vi "ExternalSetParam.vi"(0 "reference":refnum<class "ClassNode.lvclass">, 1 "setParameter":T2, 2 "string":string, 3 "position":T1 {"y" format="%.2f"; "x" format="%.2f"}, 4 "Boolean":bool, 5 "error in (no error)":errorcluster, 7 "ClassPath":path) -> (14 "reference out":refnum<class "ClassNode.lvclass">, 19 "error out":errorcluster)   [LabVIEW 2014, in "ClassNode.lvclass"]
doc: "Sets parameter externaly.\nPossible to set Name,Attrib,Methods and Position"
uses:
  <resource>/Framework/Providers/Open_GDS/UML/ClassNode_class/ClassNode.lvclass
  <resource>/Framework/Providers/Open_GDS/UML/ClassNode_class/ExternalSetTypes.ctl
  <resource>/Framework/Providers/Open_GDS/UML/General/Point/Point Point2D.ctl
  <resource>/Framework/Providers/Open_GDS/UML/MultiLineString_class/MultiLineString.lvclass
  <resource>/Framework/Providers/Open_GDS/UML/RectangularNode_class/RectangularNode.lvclass
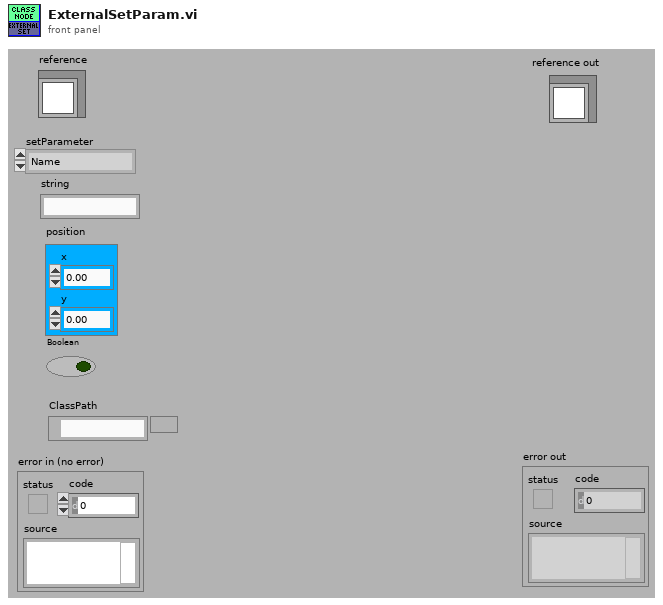
[diagram p1: front panel]
types:
  T1 = typedef "Point Point2D.ctl" = cluster{"x":dbl, "y":dbl}
  T2 = typedef "ClassNode.lvclass/ExternalSetTypes.ctl" = enum16{"Name", "Attributes", "Methods", "Position", "ShowMethods", "ShowAttributes", "ClassPath"}
  T3 = typedef "ClassNode.lvclass/ObjectAttributes.ctl" = cluster{"midHeight":dbl, "botHeight":dbl, "name":refnum<class "MultiLineString.lvclass">, "attributes":refnum<class "MultiLineString.lvclass">, "methods":refnum<class "MultiLineString.lvclass">, "DEFAULT_COMPARTMENT_HEIGHT":i32, "DEFAULT_WIDTH":i32, "DEFAULT_HEIGHT":i32, "showMethods":bool, "showAttributes":bool, "ClassPath":path}
  T4 = typedef "RectangularNode.lvclass/ObjectAttributes.ctl" = cluster{"bounds":T5}
  T5 = typedef "Rectangle Rectangle2D.ctl" = cluster{"x":dbl, "y":dbl, "width":dbl, "height":dbl}
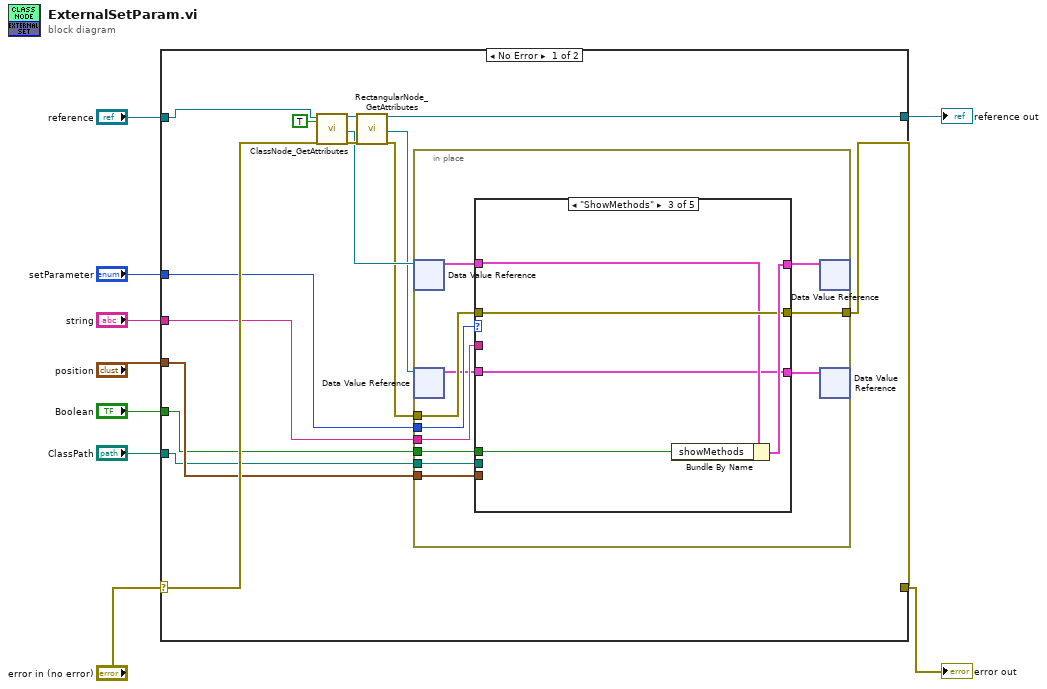
[diagram p0: block diagram]
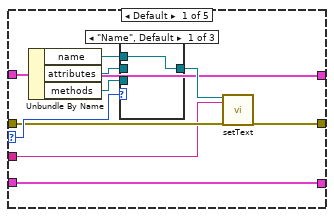
[diagram p2: hidden frame]
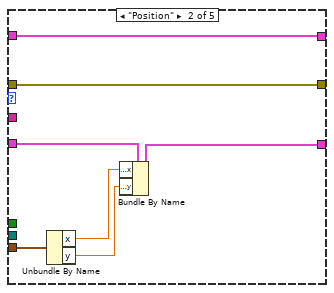
[diagram p5: hidden frame]
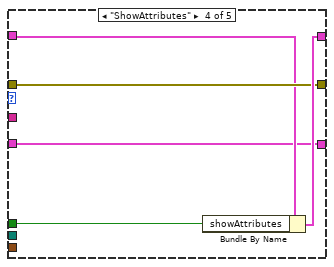
[diagram p6: hidden frame]
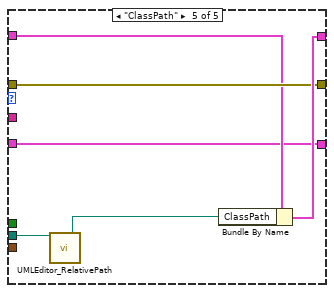
[diagram p7: hidden frame]
diagram:
  n1 = case shown="No Error" "error in (no error)" {
    selector: "error in (no error)" -> [w21 w72]
    tunnel: "reference" -> [w24 w73]
    tunnel: [w23 w72] -> w7
    tunnel: [w22 w73] -> w6
    tunnel: "setParameter" -> [w15 _]
    tunnel: "position" -> [w14 _]
    tunnel: "string" -> [w12 _]
    tunnel: "Boolean" -> [w11 _]
    tunnel: "ClassPath" -> [w10 _]
    frame No Error {
      n2 = call <resource>:"ClassNode_GetAttributes.vi"("reference in"=w24, "OnlyGetDvrReference(False)"=TRUE, "error in (no error)"=w21) -> ("reference out"=w19:refnum<class "ClassNode.lvclass">, "DataRef"=w17:refnum<data-value>, "error out"=w18:errorcluster)  [unwired: 13 in, 1 out]
      n3 = call <resource>:"RectangularNode_GetAttributes.vi"("reference in"=w19, "error in (no error)"=w18) -> ("reference out"=w22:refnum<class "ClassNode.lvclass">, "DataRef"=w16:refnum<data-value>, "error out"=w13:errorcluster)  [unwired: 14 in, 1 out]
      n4 = in-place {
        in-place-border: w15 -> [w35]
        in-place-border: w14 -> [w34]
        in-place-border: w13 -> [w33]
        in-place-border: w12 -> [w32]
        in-place-border: w11 -> [w31]
        in-place-border: w10 -> [w30]
        in-place-border: [w27] -> w23
        n5 = in-place-dvr #1(w17) -> (w29:T3)  [unwired: 1 out]
        n6 = in-place-dvr #2(w16) -> (w28:T4)  [unwired: 1 out]
        n7 = case shown="\"ShowMethods\"" w35 {
          selector: w35 -> [w45 _ _ _ _]
          tunnel: [w37 w49 w60 w65 w71] -> w26
          tunnel: w34 -> [_ w55 _ _ _]
          tunnel: w33 -> [w44 w52 w59 w64 w70]
          tunnel: [w43 w52 w59 w64 w70] -> w27
          tunnel: w32 -> [w42 _ _ _ _]
          tunnel: w31 -> [_ _ w58 w63 _]
          tunnel: w30 -> [_ _ _ _ w68]
          tunnel: w29 -> [w37 w49 w57 w62 w67]
          tunnel: w28 -> [w36 w51 w56 w61 w66]
          tunnel: [w36 w50 w56 w61 w66] -> w25
          frame Default {
            n8 = Unbundle By Name(w37) -> ("name"=w41:refnum<class "MultiLineString.lvclass">, "attributes"=w39:refnum<class "MultiLineString.lvclass">, "methods"=w38:refnum<class "MultiLineString.lvclass">)
            n9 = case shown="\"Name\", Default" w45 {
              tunnel: w41 -> [w46 _ _]
              tunnel: [w46 w47 w48] -> w40
              tunnel: w39 -> [_ w47 _]
              tunnel: w38 -> [_ _ w48]
              frame "Name", Default {
              }
              frame "Attributes" {
              }
              frame "Methods" {
              }
            }
            n10 = call-dynamic "setText.vi"("reference"=w40, "text"=w42, "error in (no error)"=w44) -> ("error out"=w43:errorcluster)  [unwired: 16 out]
          }
          frame "Position" {
            n11 = Unbundle By Name(w55) -> ("x"=w54:dbl, "y"=w53:dbl)
            n12 = Bundle By Name(cluster=w51, "bounds.x"=w54, "bounds.y"=w53) -> (w50:T4)
          }
          frame "ShowMethods" {
            n13 = Bundle By Name(cluster=w57, "showMethods"=w58) -> (w60:T3)
          }
          frame "ShowAttributes" {
            n14 = Bundle By Name(cluster=w62, "showAttributes"=w63) -> (w65:T3)
          }
          frame "ClassPath" {
            n15 = call <resource>:"UMLEditor_RelativePath.vi"("Path In"=w68) -> ("ConvertToRelativePath(If possible)"=w69:path)  [unwired: 1 in, 17 out]
            n16 = Bundle By Name(cluster=w67, "ClassPath"=w69) -> (w71:T3)
          }
        }
        n17 = in-place-dvr #1(w26) -> ()  [unwired: 2 out]
        n18 = in-place-dvr #2(w25) -> ()  [unwired: 2 out]
      }
    }
    frame Error {
    }
  }
  "reference out" <- w6
  "error out" <- w7
